vi "basic-state-machine.vi"(0 "Cluster in":refnum<vi>, 1 "Cluster 2":T3, 2 "InputData 3":refnum<vi>, 3 "Cluster 4":T2, 4 "Speaker":refnum<vi>, 5 "Lickometer 2":refnum<vi>, 6 "InputData 2":refnum<vi>, 8 "Lickometer 3":refnum<vi>, 9 "Lickometer":refnum<vi>, 10 "Time 3":refnum<vi>, 11 "InputData":refnum<vi>, 12 "Time 2":refnum<vi>, 13 "Speaker 2":refnum<vi>, 14 "InputData 4":refnum<vi>, 15 "Time":refnum<vi>, 16 "Lickometer 4":refnum<vi>, 17 "all rows":i64[](array[numeric]), 18 "Enum in":T1) -> (20 "Cluster 3":T3, 21 "String":string, 22 "Boolean":bool, 23 "Cluster":T2, 24 "Enum out":T1)   [LabVIEW 2015]
uses:
  states-enum.ctl
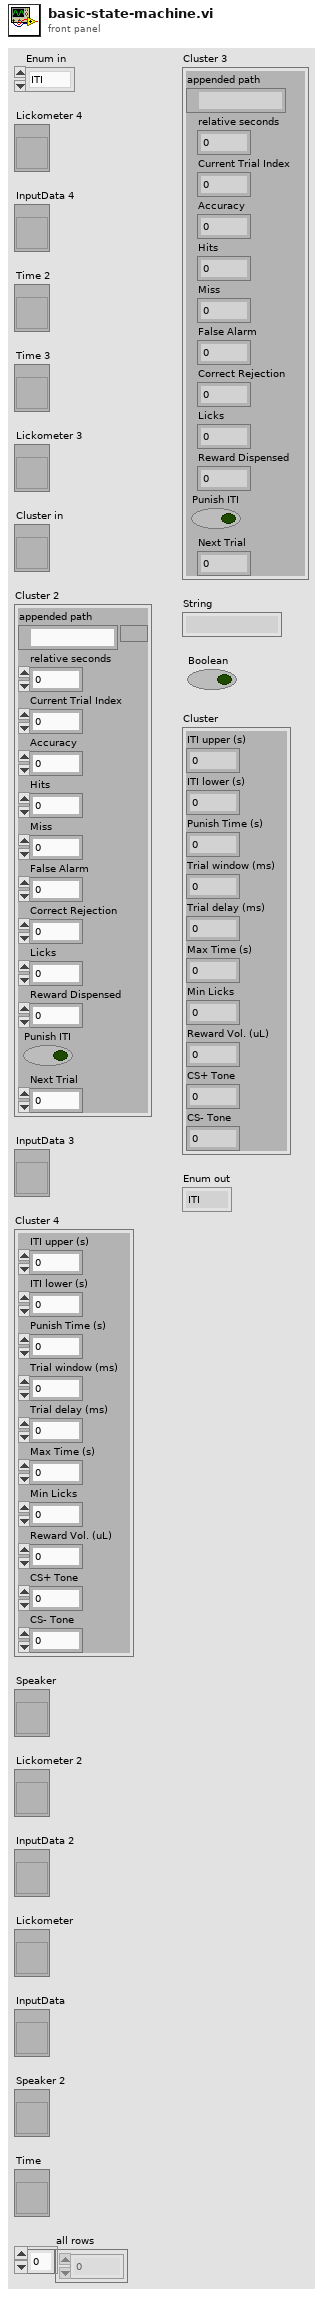
[diagram p1: front panel]
types:
  T1 = typedef "states-enum.ctl" = enum16{"ITI", "Trial", "Stop"}
  T2 = cluster{"ITI upper (s)":dbl, "ITI lower (s)":dbl, "Punish Time (s)":dbl, "Trial window (ms)":dbl, "Trial delay (ms)":dbl, "Max Time (s)":dbl, "Min Licks":i32, "Reward Vol. (uL)":dbl, "CS+ Tone":i32, "CS- Tone":i32}
  T3 = cluster{"appended path":path, "relative seconds":dbl, "Current Trial Index":i32, "Accuracy":dbl, "Hits":i32, "Miss":i32, "False Alarm":i32, "Correct Rejection":i32, "Licks":i32, "Reward Dispensed":dbl, "Punish ITI":bool, "Next Trial":i32}
  T4 = cluster{"Trial Hit":bool, "Trial Miss":bool, "Trial FA":bool, "Trial CR":bool, "Skip Receiving":bool}
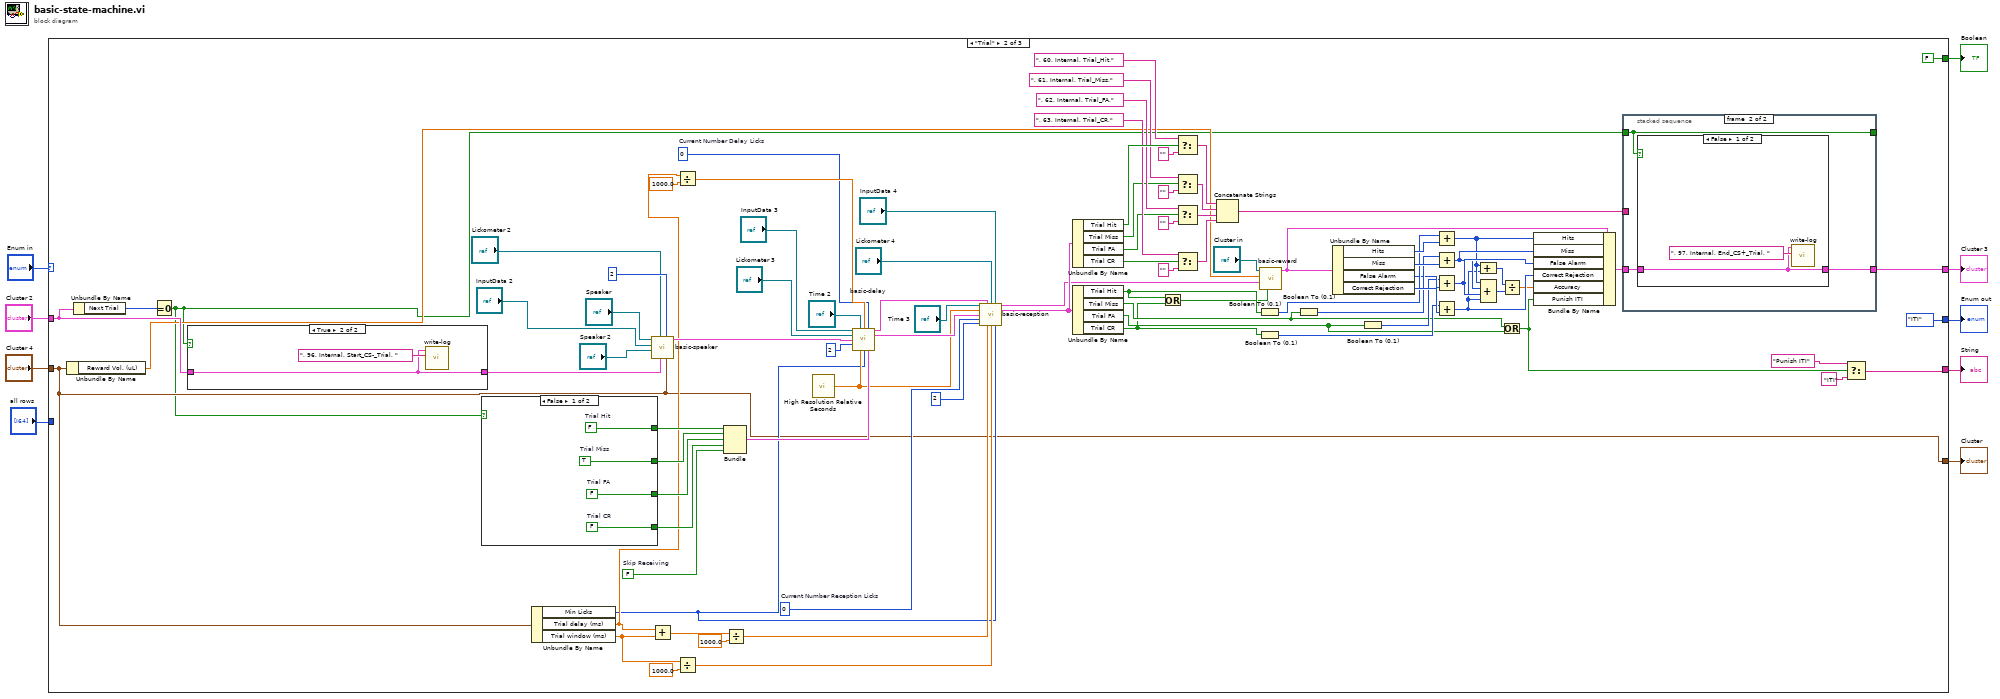
[diagram p0: block diagram]
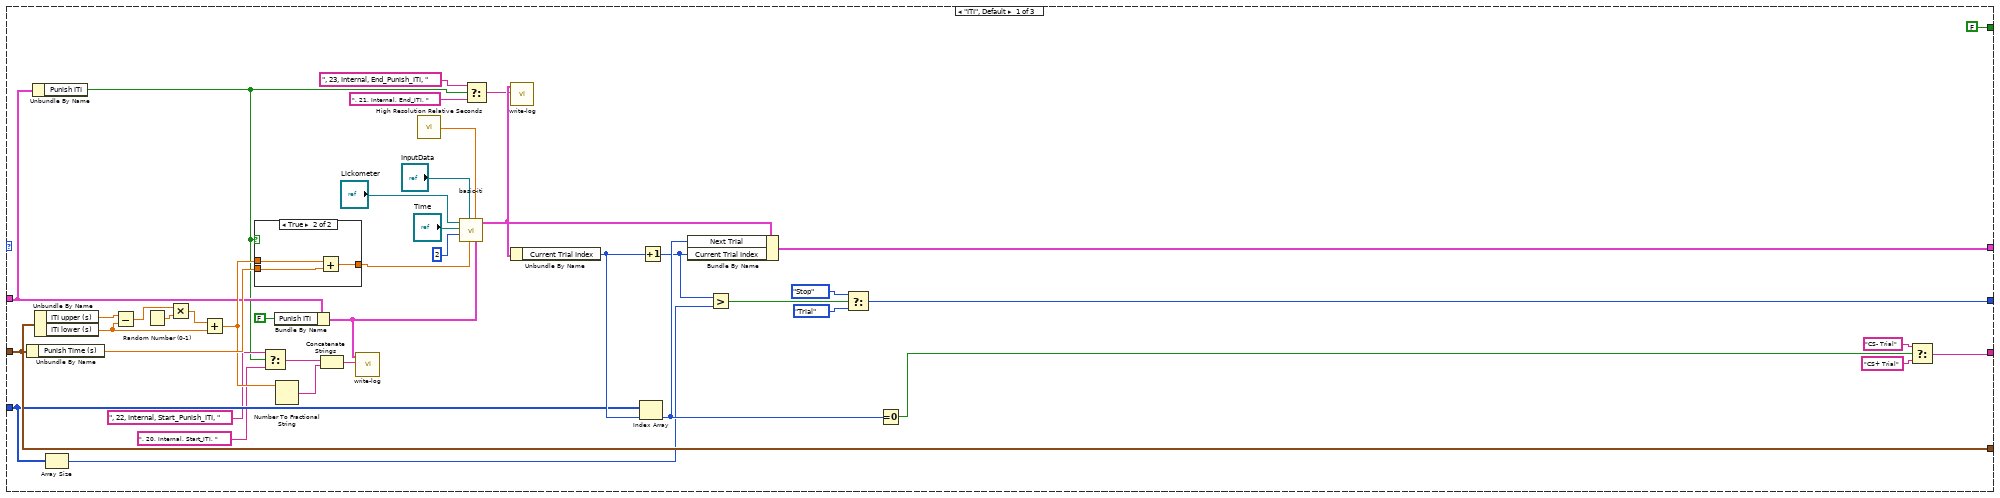
[diagram p2: hidden frame]
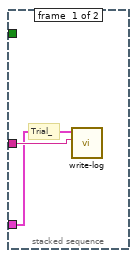
[diagram p4: hidden frame]
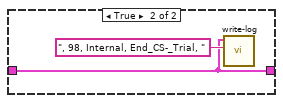
[diagram p5: hidden frame]
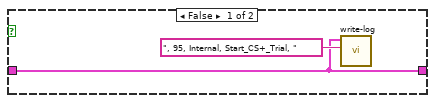
[diagram p6: hidden frame]
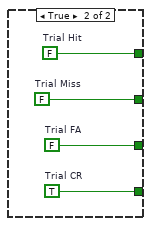
[diagram p7: hidden frame]
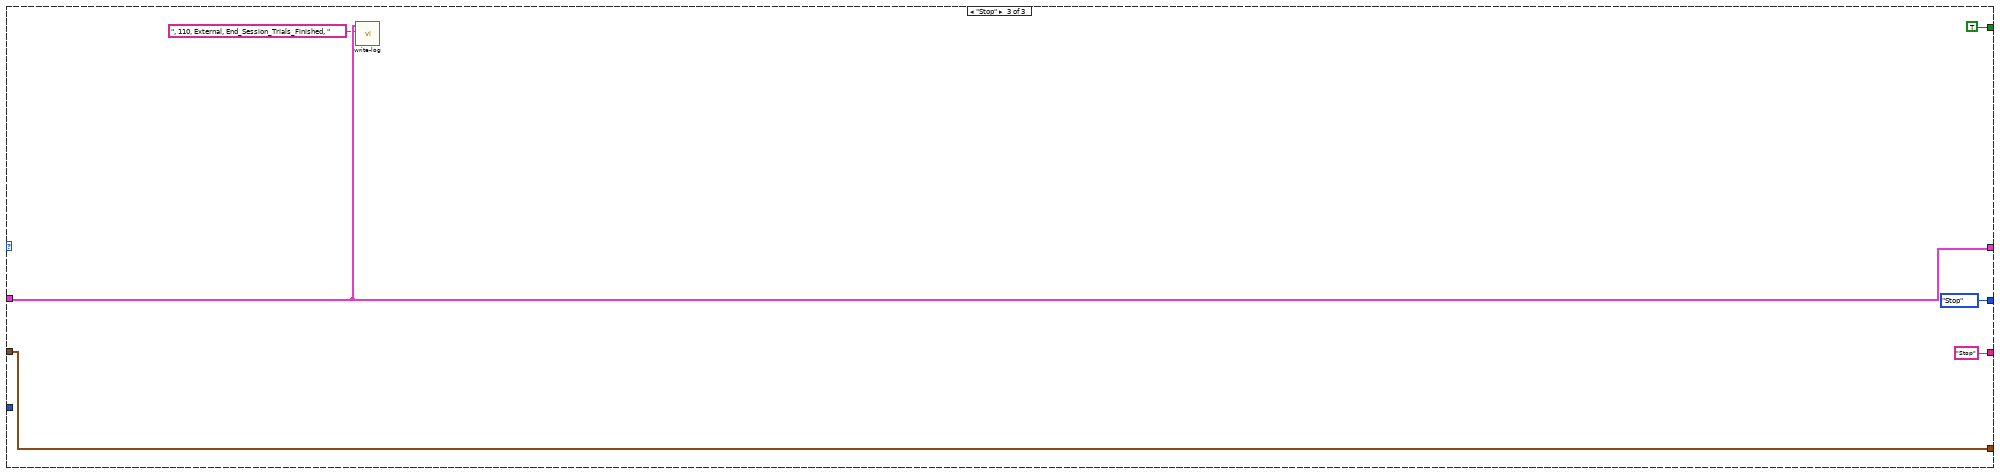
[diagram p8: hidden frame]
diagram:
  n1 = case shown="\"Trial\"" "Enum in" {
    tunnel: [w27 states-enum."ITI" states-enum."Stop"] -> w1
    tunnel: [FALSE FALSE TRUE] -> w2
    tunnel: "all rows" -> [w32 _ _]
    tunnel: [w36 w107 "Stop"] -> w4
    tunnel: "Cluster 4" -> [w35 w73 w172]
    tunnel: [w41 w72 w168] -> w6
    tunnel: "Cluster 2" -> [w26 w76 w168]
    tunnel: [w35 w73 w172] -> w8
    frame "ITI", Default {
      n2 = Unbundle By Name(w35) -> ("Punish Time (s)"=w34:dbl)
      n3 = Unbundle By Name(w26) -> ("Punish ITI"=w17:bool)
      n4 = Unbundle By Name(w35) -> ("ITI upper (s)"=w44:dbl, "ITI lower (s)"=w48:dbl)
      n5 = Array Size(array=w32) -> (size(s)=w31:i32)
      n6 = Subtract(x=w44, y=w48) -> (x-y=w45:dbl)
      n7 = Random Number (0-1)() -> (number: 0 to 1=w46:dbl)
      n8 = Multiply(x=w45, y=w46) -> (x*y=w47:dbl)
      n9 = Add(x=w47, y=w48) -> (x+y=w33:dbl)
      n10 = case shown="True" w17 {
        tunnel: w33 -> [w52 w55]
        tunnel: [w52 w54] -> w15
        tunnel: w34 -> [_ w53]
        frame False {
        }
        frame True {
          n11 = Add(x=w55, y=w53) -> (x+y=w54:dbl)
        }
      }
      n12 = Select(t=", 22, Internal, Start_Punish_ITI, " ("text"), s=w17, f=", 20, Internal, Start_ITI, " ("text")) -> (s? t:f=w21:string)
      n13 = Bundle By Name(cluster=w26, "Punish ITI"=FALSE) -> (w25:T3)
      n14 = Number To Fractional String(number=w33) -> (F-format string=w50:string)  [unwired: 3 in]
      n15 = Concatenate Strings(w21, w50) -> (w49:string)
      n16 = call "write-log.vi"("Write Text"=w49, "Internal Cluster"=w25) -> ()  [unwired: 10 in]
      n17 = call <vilib>:"High Resolution Relative Seconds.vi"() -> ("relative seconds"=w16:dbl)
      n18 = call "basic-iti.vi"("Cluster"=w25, "relative seconds"=w16, "Numeric"=w15, "reference"="InputData", "Period"=i64 2, "reference 2"="Time", "Cluster in"="Lickometer") -> ("Cluster 2"=w42:T3)  [unwired: 4 in]
      n19 = Select(t=", 23, Internal, End_Punish_ITI, " ("text"), s=w17, f=", 21, Internal, End_ITI, " ("text")) -> (s? t:f=w20:string)
      n20 = call "write-log.vi"("Write Text"=w20, "Internal Cluster"=w42) -> ()  [unwired: 10 in]
      n21 = Unbundle By Name(w42) -> ("Current Trial Index"=w43:i32)
      n22 = Index Array(array=w32, index=w43) -> (element=w40:i64)
      n23 = Increment(x=w43) -> (x+1=w30:i32)
      n24 = Bundle By Name(cluster=w42, "Next Trial"=w40, "Current Trial Index"=w30) -> (w41:T3)
      n25 = Greater?(x=w30, y=w31) -> (0:w29:bool)
      n26 = Select(t=states-enum."Stop", s=w29, f=states-enum."Trial") -> (s? t:f=w27:T1)
      n27 = Equal To 0?(x=w40) -> (x = 0?=w39:bool)
      n28 = Select(t="CS- Trial", s=w39, f="CS+ Trial") -> (s? t:f=w36:string)
    }
    frame "Trial" {
      w78 = 0  # Current Number Reception Licks
      w79 = 0  # Current Number Delay Licks
      w81 = FALSE  # Skip Receiving
      n29 = Unbundle By Name(w73) -> ("Reward Vol. (uL)"=w74:dbl)
      n30 = Unbundle By Name(w76) -> ("Next Trial"=w132:i32)
      n31 = Equal To 0?(x=w132) -> (x = 0?=w70:bool)
      n32 = case shown="True" w70 {
        tunnel: w76 -> [w155 w157]
        tunnel: [w155 w157] -> w75
        frame False {
          n33 = call "write-log.vi"("Write Text"=", 95, Internal, Start_CS+_Trial, " ("text"), "Internal Cluster"=w155) -> ()  [unwired: 10 in]
        }
        frame True {
          n34 = call "write-log.vi"("Write Text"=", 96, Internal, Start_CS-_Trial, " ("text"), "Internal Cluster"=w157) -> ()  [unwired: 10 in]
        }
      }
      n35 = case shown="False" w70 {
        tunnel: [w162 w166] -> w137
        tunnel: [w161 w165] -> w136
        tunnel: [w160 w164] -> w135
        tunnel: [w159 w163] -> w134
        frame False {
          w159 = FALSE  # Trial CR
          w160 = FALSE  # Trial FA
          w161 = TRUE  # Trial Miss
          w162 = FALSE  # Trial Hit
        }
        frame True {
          w163 = TRUE  # Trial CR
          w164 = FALSE  # Trial FA
          w165 = FALSE  # Trial Miss
          w166 = FALSE  # Trial Hit
        }
      }
      n36 = Unbundle By Name(w73) -> ("Min Licks"=w77:i32, "Trial delay (ms)"=w109:dbl, "Trial window (ms)"=w101:dbl)
      n37 = call "basic-speaker.vi"("Cluster"=w73, "Period"=i64 2, "Cluster 2"=w75, "Lickometer"="Lickometer 2", "Speaker in"="Speaker 2", "reference"="InputData 2", "Cluster in"="Speaker") -> ("Cluster 3"=w138:T3)  [unwired: 4 in]
      n38 = Add(x=w109, y=w101) -> (x+y=w108:dbl)
      n39 = Divide(x=w109, y=1000.0) -> (x/y=w142:dbl)
      n40 = Divide(x=w101, y=1000.0) -> (x/y=w102:dbl)
      n41 = Bundle("Trial Hit"=w137, "Trial Miss"=w136, "Trial FA"=w135, "Trial CR"=w134, "Skip Receiving"=w81) -> (w133:T4)  [unwired: 1 in]
      n42 = Divide(x=w108, y=1000.0) -> (x/y=w140:dbl)
      n43 = call <vilib>:"High Resolution Relative Seconds.vi"() -> ("relative seconds"=w110:dbl)
      n44 = call "basic-delay.vi"("Cluster in"="InputData 3", "reference in"="Time 2", "Numeric"=w142, "Current Number Delay Licks"=w79, "Lickometer"="Lickometer 3", "Cluster 3"=w138, "Period"=i64 2, "relative seconds"=w110, "Min Licks"=w77, "Cluster 2"=w133) -> ("Cluster 4"=w141:T3, "Cluster"=w131:T4)  [unwired: 4 in]
      n45 = call "basic-reception.vi"("Digital in"="Time 3", "Cluster 5"=w141, "Lickometer"="Lickometer 4", "reference in"="InputData 4", "relative seconds"=w110, "Cluster in"=w131, "Current Number Reception Licks"=w78, "Period"=i64 2, "Numeric 2"=w140, "Numeric"=w102, "Min Licks"=w77) -> ("Cluster 4"=w80:T3, "Cluster out"=w100:T4)  [unwired: 3 in]
      n46 = Unbundle By Name(w100) -> ("Trial Hit"=w99:bool, "Trial Miss"=w90:bool, "Trial FA"=w89:bool, "Trial CR"=w88:bool)
      n47 = Unbundle By Name(w100) -> ("Trial Hit"=w113:bool, "Trial Miss"=w115:bool, "Trial FA"=w114:bool, "Trial CR"=w112:bool)
      n48 = Or(x=w113, y=w112) -> (x .or. y?=w111:bool)
      n49 = Select(t=", 60, Internal, Trial_Hit," ("text"), s=w99, f="") -> (s? t:f=w87:string)
      n50 = Select(t=", 61, Internal, Trial_Miss," ("text"), s=w90, f="") -> (s? t:f=w86:string)
      n51 = Select(t=", 62, Internal, Trial_FA," ("text"), s=w89, f="") -> (s? t:f=w85:string)
      n52 = Select(t=", 63, Internal, Trial_CR," ("text"), s=w88, f="") -> (s? t:f=w84:string)
      n53 = Concatenate Strings(w87, w86, w85, w84) -> (w83:string)
      n54 = Boolean To (0,1)(Boolean=w113) -> (0, 1=w125:i16)
      n55 = Boolean To (0,1)(Boolean=w112) -> (0, 1=w127:i16)
      n56 = call "basic-reward.vi"("Boolean"=w111, "Cluster 5"=w80, "Reward Vol. (uL)"=w74, "Cluster in"="Cluster in") -> ("Cluster 4"=w71:T3)  [unwired: 7 in]
      n57 = Boolean To (0,1)(Boolean=w115) -> (0, 1=w126:i16)
      n58 = Unbundle By Name(w71) -> ("Hits"=w130:i32, "Miss"=w129:i32, "False Alarm"=w124:i32, "Correct Rejection"=w128:i32)
      n59 = Boolean To (0,1)(Boolean=w114) -> (0, 1=w123:i16)
      n60 = Add(x=w125, y=w130) -> (x+y=w120:i32)
      n61 = Add(x=w126, y=w129) -> (x+y=w121:i32)
      n62 = Add(x=w123, y=w124) -> (x+y=w122:i32)
      n63 = Add(x=w127, y=w128) -> (x+y=w119:i32)
      n64 = Compound Arithmetic op=ADD(w120, w119) -> (w118:i32)
      n65 = Compound Arithmetic op=ADD(w120, w121, w122, w119) -> (w117:i32)
      n66 = Divide(x=w118, y=w117) -> (x/y=w116:dbl)
      n67 = Or(x=w115, y=w114) -> (x .or. y?=w106:bool)
      n68 = Bundle By Name(cluster=w71, "Hits"=w120, "Miss"=w121, "False Alarm"=w122, "Correct Rejection"=w119, "Accuracy"=w116, "Punish ITI"=w106) -> (w82:T3)
      n69 = stacked-sequence {
        tunnel: w83 -> [w147 _]
        tunnel: w82 -> [w146 w150]
        tunnel: [_ w149] -> w72
        tunnel: [_ w148] -> _
        tunnel: w70 -> [_ w148]
        frame #0 {
          # "Trial_"
          n70 = call "write-log.vi"("Write Text"=w147, "Internal Cluster"=w146) -> ()  [unwired: 10 in]
        }
        frame #1 {
          n71 = case shown="False" w148 {
            tunnel: w150 -> [w151 w153]
            tunnel: [w151 w153] -> w149
            frame False {
              n72 = call "write-log.vi"("Write Text"=", 97, Internal, End_CS+_Trial, " ("text"), "Internal Cluster"=w151) -> ()  [unwired: 10 in]
            }
            frame True {
              n73 = call "write-log.vi"("Write Text"=", 98, Internal, End_CS-_Trial, " ("text"), "Internal Cluster"=w153) -> ()  [unwired: 10 in]
            }
          }
        }
      }
      n74 = Select(t="Punish ITI", s=w106, f="ITI") -> (s? t:f=w107:string)
    }
    frame "Stop" {
      n75 = call "write-log.vi"("Write Text"=", 110, External, End_Session_Trials_Finished, " ("text"), "Internal Cluster"=w168) -> ()  [unwired: 10 in]
    }
  }
  "Cluster" <- w8
  "Cluster 3" <- w6
  "String" <- w4
  "Boolean" <- w2
  "Enum out" <- w1
